vi "Close2001.vi"   [LabVIEW 2013]
uses:
  <vilib>/Heliosphere Research LLC/Advanced Plotting Toolkit/typedefs/PlotID.ctl
  <vilib>/Heliosphere Research LLC/Advanced Plotting Toolkit/Advanced Plotting Toolkit.lvlib
types:
  T1 = typedef "Advanced Plotting Toolkit.lvlib/PlotID.ctl" = i32
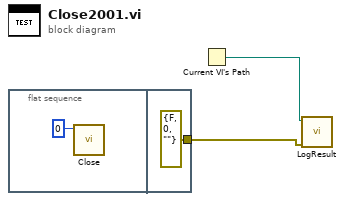
[diagram p0: block diagram]
diagram:
  n1 = flat-sequence {
    tunnel: [errorcluster {"status"=FALSE, "code"=0, "source"=""} ("Test Result")] -> w1
    frame #0 {
      n2 = call <vilib>:"Close.vi"("Plot ID"=T1 0) -> ()  [unwired: 11 in]
    }
    frame #1 {
    }
  }
  n3 = Current VI's Path() -> (path=w2:path)
  n4 = call "LogResult.vi"("Test Result"=w1, "VI Path"=w2) -> ()  [unwired: 10 in]
